vi "send_book.vi"(8 "error in (no error)":errorcluster, 10 "book text":string, 11 "client in":refnum<class "client.lvclass">) -> (0 "error out":errorcluster, 3 "client out":refnum<class "client.lvclass">)   [LabVIEW 2020, in "client.lvclass"]
uses:
  client.lvclass
  client.lvclass/client.ctl
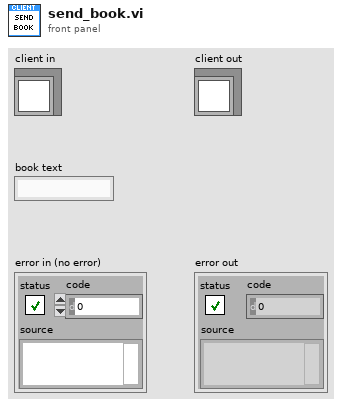
[diagram p1: front panel]
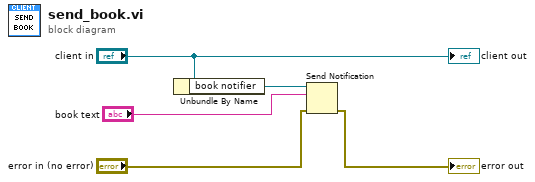
[diagram p0: block diagram]
diagram:
  n1 = Unbundle By Name("client in") -> ("book notifier"=w4:refnum<notifier>)
  n2 = Send Notification(notification="book text", notifier=w4, error in (no error)="error in (no error)") -> (error out=→"error out":errorcluster)  [unwired: 1 out]
  "client out" <- "client in"
